vi "Password_Popup.vi"(0 "Application_Directory":path, 11 "Error_In":errorcluster) -> (15 "Error_Out":errorcluster)   [LabVIEW 2023]
doc: "This is a VI work as one of the front panel of the Game, asking the user Password for the game to start up."
uses:
  Controls/Bool_Button.ctl
  <vilib>/Utility/miscctls.llb/LVTextColorsTypeDef.ctl
  Controls/State.ctl
panel:
  in  "Close?":T1
  in  "Password_Enter?":T1
  in  "Enter_Password":string caption="Enter Password"
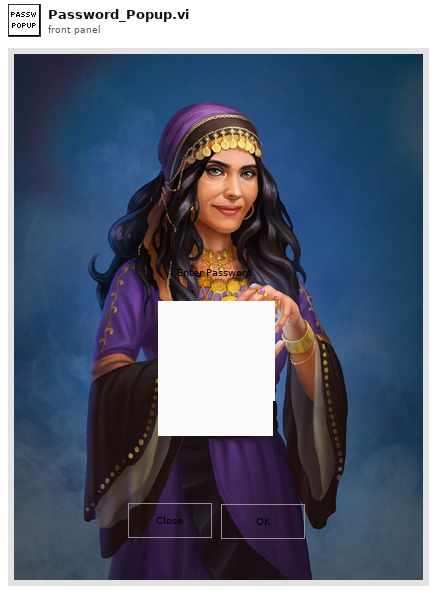
[diagram p1: front panel]
types:
  T1 = typedef "Bool_Button.ctl" = bool
  T2 = enum32{"Invalid", "Standard", "Closed", "Hidden", "Minimized", "Maximized"}
  T3 = typedef "LVTextColorsTypeDef.ctl" = cluster{"Text Color":u32, "Background Color":u32}
  T4 = typedef "State.ctl" = enum16{"Close", "Password_Popup", "Start_Popup", "Wizard_Msg", "Get_Name_DoB", "Lucky_Number", "Q-1", "Q-2", "Q-3", "Nature_of_the_Person"}
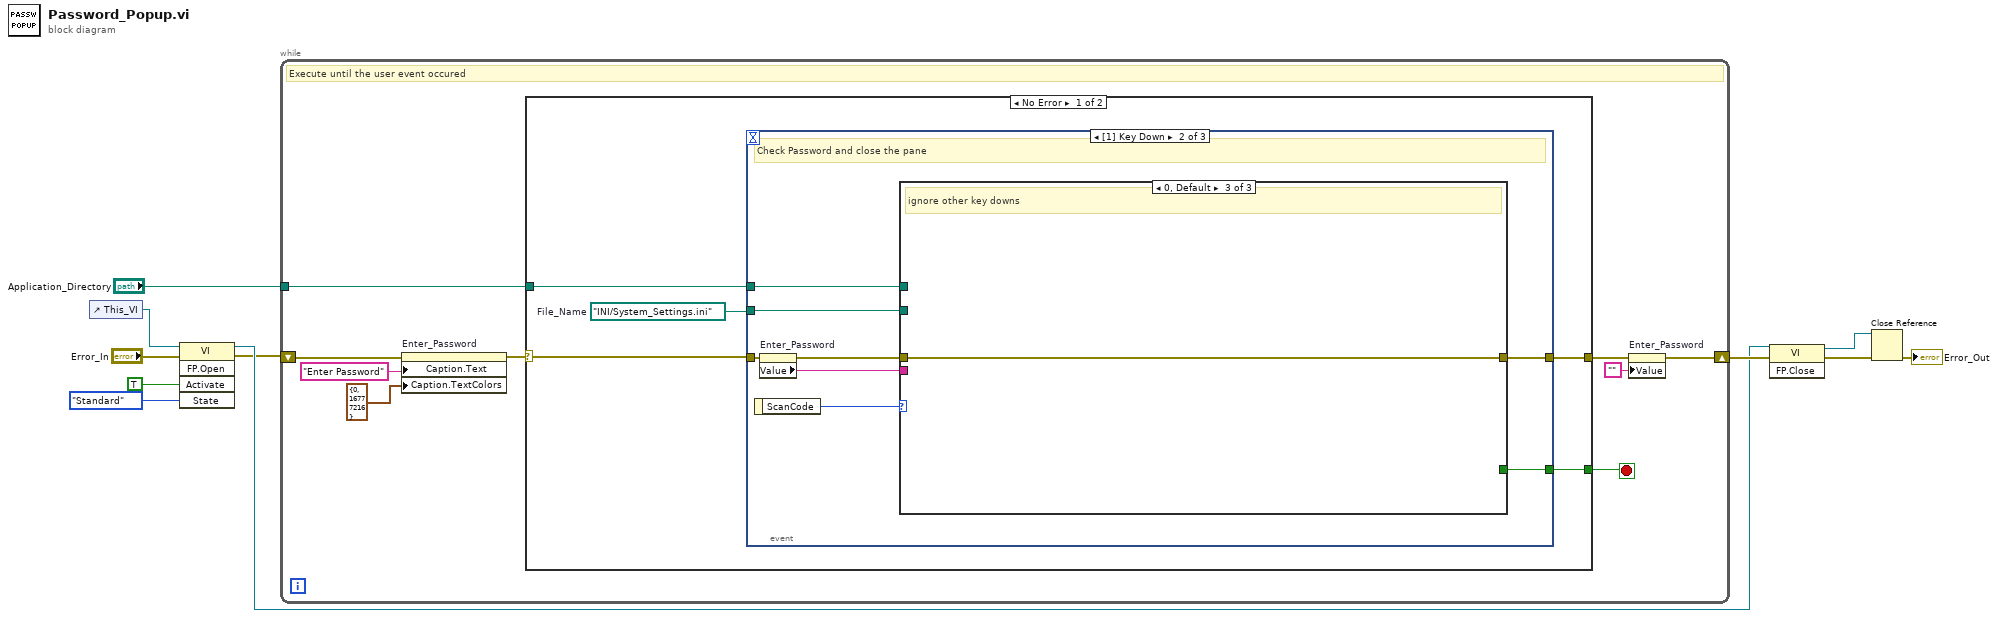
[diagram p0: block diagram]
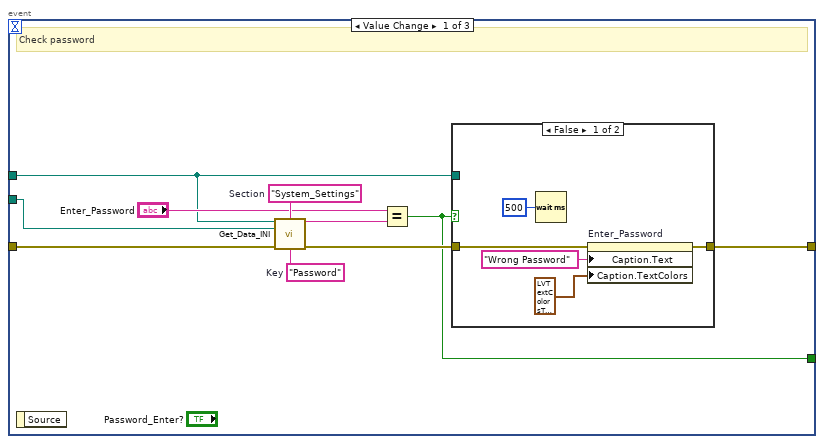
[diagram p2: hidden frame]
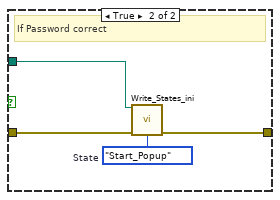
[diagram p3: hidden frame]
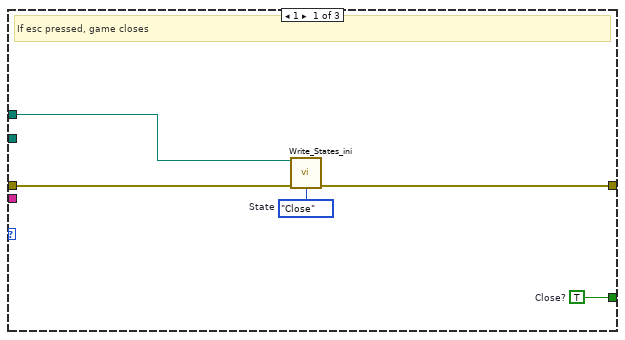
[diagram p4: hidden frame]
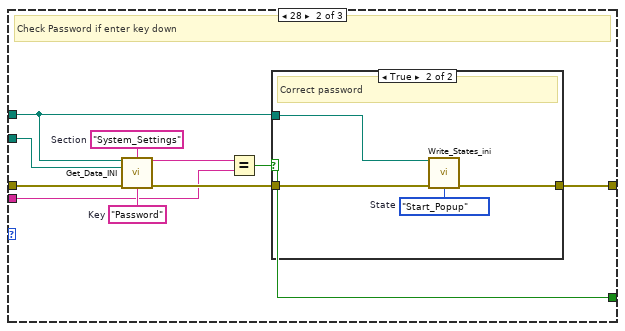
[diagram p5: hidden frame]
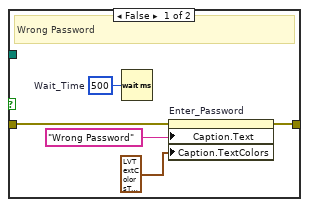
[diagram p6: hidden frame]
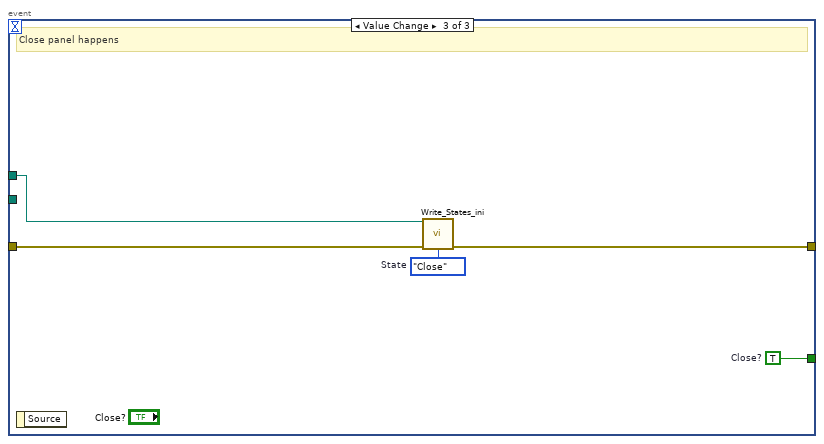
[diagram p7: hidden frame]
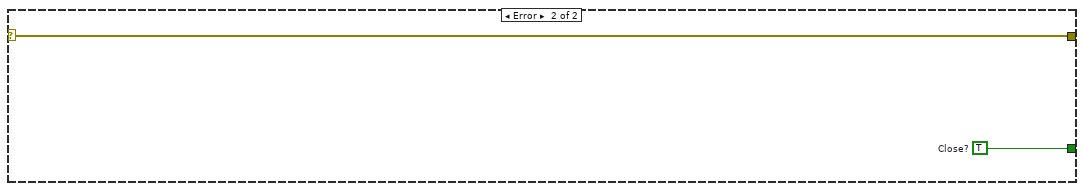
[diagram p8: hidden frame]
diagram:
  n1 = control-ref of="This_VI"() -> (w9:refnum<vi>)
  n2 = invoke class="VI" method="FP.Open"(reference=w9, error in="Error_In", "Activate"=TRUE ("Activate?"), "State"=T2."Standard") -> (reference out=w8:refnum<vi>, error out=w1:errorcluster)  [unwired: 1 in, 3 out]
  n3 = while {
    tunnel: "Application_Directory" -> [w20]
    shift-right: [w12] -> w11
    shift-left: w1 -> [w17]
    stop <- w15 stop-if-true
    # "Execute until the user event occured"
    n4 = property on="Enter_Password" class="Str"(error in=w17, "Caption.Text"="Enter Password", "Caption.TextColors"=T3 {"Text Color"=0, "Background Color"=16777216} ("Caption.Text Colors")) -> (error out=w16:errorcluster)  [unwired: 1 in, 1 out]
    n5 = case shown="No Error" w16 {
      selector: w16 -> [w25 w84]
      tunnel: [w24 w84] -> w13
      tunnel: w20 -> [w23 _]
      tunnel: [w22 w83] -> w15
      frame No Error {
        w21 = path "INI/System_Settings.ini"  # File_Name
        n6 = event shown="[1] Key Down" {
          selector: _ -> [_ _ _]
          dyn-events: _ -> [_ _ _]
          timeout: _ -> [_ _ _]
          tunnel: w25 -> [w32 w50 w80]
          tunnel: [w30 w51 w79] -> w24
          tunnel: w23 -> [w26 w52 w78]
          tunnel: [w27 w45 w82] -> w22
          tunnel: w21 -> [w28 w48 _]
          event Value Change {
            w35 = "Password"  # Key
            w34 = "System_Settings"  # Section
            # "Check password"
            n7 = event-data() -> ()  [unwired: 1 in, 1 out]
            n8 = call "Get_Data_INI.vi"("Application_Directory"=w26, "Section"=w34, "File_Name"=w28, "Error_In"=w32, "Key"=w35) -> ("Data"=w33:string, "Error_Out"=w31:errorcluster)  [unwired: 9 in]
            n9 = Equal?(x="Enter_Password", y=w33) -> (x = y?=w27:bool)
            n10 = case shown="False" w27 {
              tunnel: w31 -> [w40 w43]
              tunnel: [w39 w42] -> w30
              tunnel: w26 -> [_ w41]
              frame False {
                n11 = Wait (ms)(milliseconds to wait=u32 500) -> ()  [unwired: 1 out]
                n12 = property on="Enter_Password" class="Str"(error in=w40, "Caption.Text"="Wrong Password", "Caption.TextColors"=T3 {"Text Color"=14421504, "Background Color"=16777216} ("Caption.Text Colors")) -> (error out=w39:errorcluster)  [unwired: 1 in, 1 out]
              }
              frame True {
                w44 = State."Start_Popup"  # State
                # "If Password correct"
                n13 = call "Write_States_ini.vi"("Application_Directory"=w41, "Error_In"=w43, "State"=w44) -> ("Error_Out"=w42:errorcluster)  [unwired: 12 in]
              }
            }
          }
          event Key Down {
            # "Check Password and close the pane"
            n14 = event-data() -> ("ScanCode"=w46:i16)  [unwired: 1 in]
            n15 = property on="Enter_Password" class="Str"(error in=w50) -> (error out=w49:errorcluster, "Value"=w47:string)  [unwired: 1 in, 1 out]
            n16 = case shown="0, Default" w46 {
              tunnel: w52 -> [w54 w59 _]
              tunnel: [w55 w63 w77] -> w51
              tunnel: w49 -> [w56 w62 w77]
              tunnel: w48 -> [_ w61 _]
              tunnel: w47 -> [_ w60 _]
              tunnel: [w57 w58 _] -> w45
              frame 1 {
                w53 = State."Close"  # State
                w57 = TRUE  # Close?
                # "If esc pressed, game closes"
                n17 = call "Write_States_ini.vi"("Application_Directory"=w54, "Error_In"=w56, "State"=w53) -> ("Error_Out"=w55:errorcluster)  [unwired: 12 in]
              }
              frame 28 {
                w67 = "Password"  # Key
                w66 = "System_Settings"  # Section
                # "Check Password if enter key down"
                n18 = call "Get_Data_INI.vi"("Application_Directory"=w59, "Section"=w66, "File_Name"=w61, "Error_In"=w62, "Key"=w67) -> ("Data"=w65:string, "Error_Out"=w64:errorcluster)  [unwired: 9 in]
                n19 = Equal?(x=w65, y=w60) -> (x = y?=w58:bool)
                n20 = case shown="True" w58 {
                  tunnel: w64 -> [w70 w76]
                  tunnel: [w71 w75] -> w63
                  tunnel: w59 -> [_ w73]
                  frame False {
                    w72 = u32 500  # Wait_Time
                    # "Wrong Password"
                    n21 = Wait (ms)(milliseconds to wait=w72) -> ()  [unwired: 1 out]
                    n22 = property on="Enter_Password" class="Str"(error in=w70, "Caption.Text"="Wrong Password", "Caption.TextColors"=T3 {"Text Color"=14421504, "Background Color"=16777216} ("Caption.Text Colors")) -> (error out=w71:errorcluster)  [unwired: 1 in, 1 out]
                  }
                  frame True {
                    w74 = State."Start_Popup"  # State
                    # "Correct password"
                    n23 = call "Write_States_ini.vi"("Application_Directory"=w73, "Error_In"=w76, "State"=w74) -> ("Error_Out"=w75:errorcluster)  [unwired: 12 in]
                  }
                }
              }
              frame 0, Default {
                # "ignore other key downs"
              }
            }
          }
          event Value Change {
            w81 = State."Close"  # State
            w82 = TRUE  # Close?
            # "Close panel happens"
            n24 = event-data() -> ()  [unwired: 1 in, 1 out]
            n25 = call "Write_States_ini.vi"("Application_Directory"=w78, "Error_In"=w80, "State"=w81) -> ("Error_Out"=w79:errorcluster)  [unwired: 12 in]
          }
        }
      }
      frame Error {
        w83 = TRUE  # Close?
      }
    }
    n26 = property on="Enter_Password" class="Str"(error in=w13, "Value"="") -> (error out=w12:errorcluster)  [unwired: 1 in, 1 out]
  }
  n27 = invoke class="VI" method="FP.Close"(reference=w8, error in=w11) -> (reference out=w7:refnum<vi>, error out=w6:errorcluster)  [unwired: 1 in, 1 out]
  n28 = Close Reference(reference=w7, error in (no error)=w6) -> (error out=→"Error_Out":errorcluster)
